vi "Read Config.vi"(6 "wait for reply (T)":bool=TRUE, 8 "error in":errorcluster) -> (0 "error out":errorcluster, 1 "timed out?":bool, 2 "Señal Digital":T1={"Puertos/Pines"="", "Puerto"="DAQSim1", "Pines"=[], "Tiempo de AQ"=0.0, "Tiempo entre AQ"=0.0}, 3 "Señal Analogica":T2={"Canal/Canales"="", "Canal"="DAQSim1", "Canales"=[], "Frecuencia de muestreo"=1000, "Numero de muestras"=1000, "Tiempo de AQ"=0.0})   [LabVIEW 2020, in "Settings.lvlib"]
doc: "Read Digital and Analog info from Data Base\n_____\nCreated using Delacor QMH Event Scripter 6.0.0.121."
uses:
  Settings.lvlib
  Aqcisition/Analog Signal Config.ctl
  Aqcisition/Digital Signal Config.ctl
  Read Config Argument--cluster.ctl
  Read Config (Reply Payload)--cluster.ctl
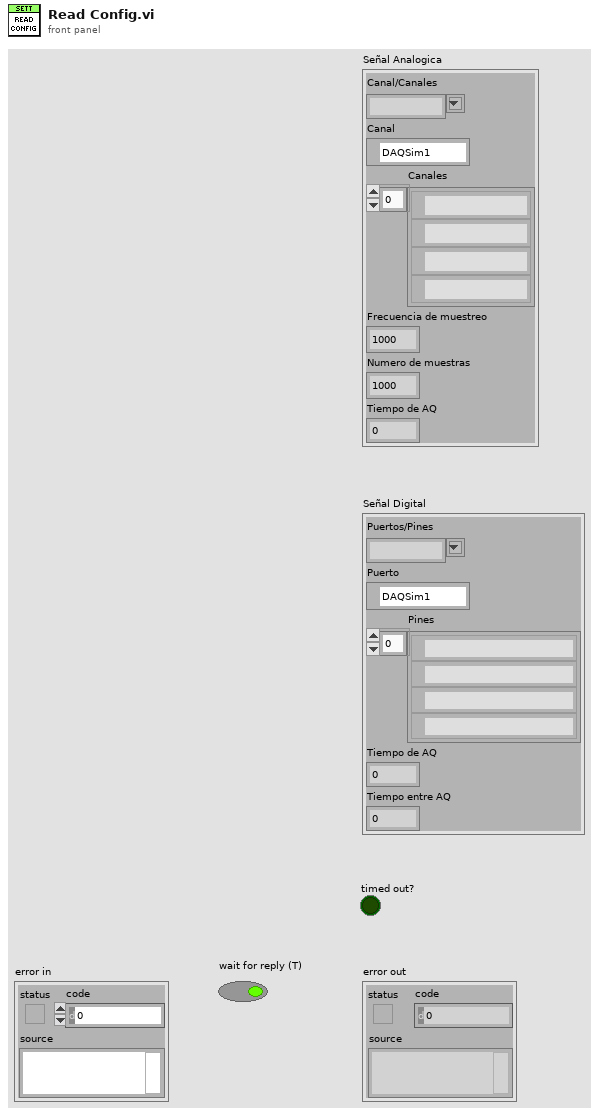
[diagram p1: front panel]
types:
  T1 = typedef "Digital Signal Config.ctl" = cluster{"Puertos/Pines":string, "Puerto":tag, "Pines":tag[], "Tiempo de AQ":dbl, "Tiempo entre AQ":dbl}
  T2 = typedef "Analog Signal Config.ctl" = cluster{"Canal/Canales":string, "Canal":tag, "Canales":tag[], "Frecuencia de muestreo":i32, "Numero de muestras":i32, "Tiempo de AQ":dbl}
  T3 = typedef "Settings.lvlib/Read Config Argument--cluster.ctl" = cluster{"Wait Notifier":refnum<notifier>, "wait for reply":bool}
  T4 = typedef "Settings.lvlib/Request Events--cluster.ctl" = cluster{"Stop Module":refnum<user-event>, "Show Panel":refnum<user-event>, "Hide Panel":refnum<user-event>, "Get Module Execution Status":refnum<user-event>, "Show Diagram":refnum<user-event>, "Save Config":refnum<user-event>, "Read Config":refnum<user-event>, "Save the config":refnum<user-event>, "Cancel config":refnum<user-event>}
  T5 = typedef "Settings.lvlib/Read Config (Reply Payload)--cluster.ctl" = cluster{"Señal Analogica":T2, "Señal Digital":T1, "Read Config_error":errorcluster}
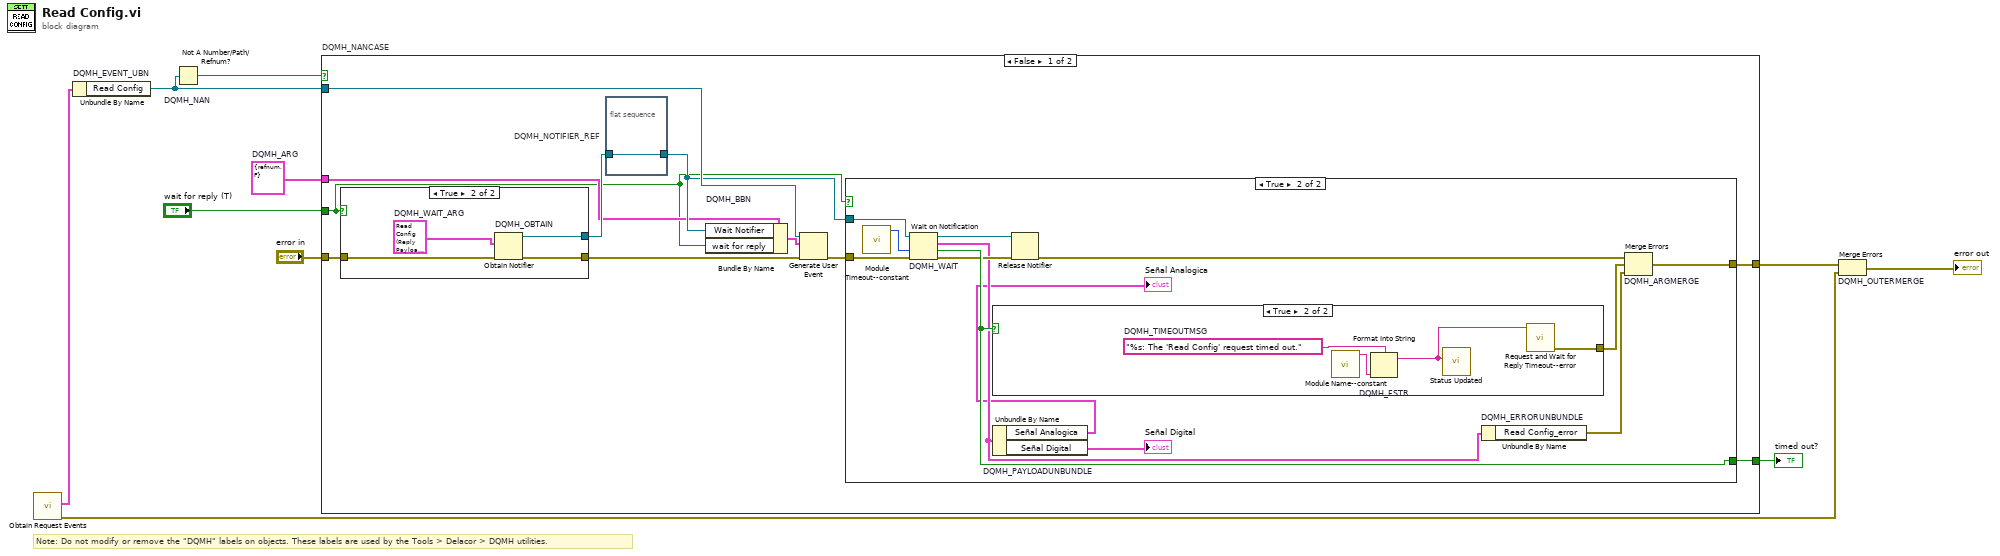
[diagram p0: block diagram]
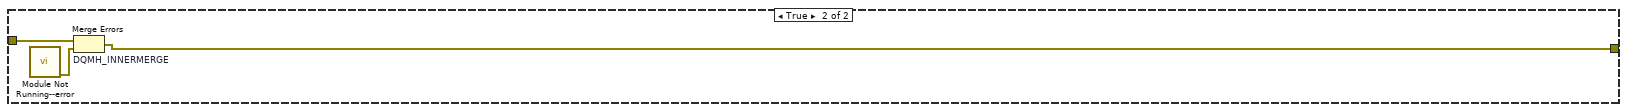
[diagram p5: hidden frame]
diagram:
  w4 = T3 {"Wait Notifier"=refnum, "wait for reply"=FALSE}  # DQMH_ARG
  # "Note: Do not modify or remove the \"DQMH\" labels on objects. These labels are used by the Tools > Delacor > DQMH utilities."
  n1 = call "Obtain Request Events.vi"() -> ("error out"=w2:errorcluster, "Settings Request Events"=w1:T4)  [unwired: 10 in]
  n2 = Unbundle By Name "DQMH_EVENT_UBN"(w1) -> ("Read Config"=w8:refnum<user-event>)
  n3 = Not A Number/Path/Refnum? "DQMH_NAN"(number/path/refnum=w8) -> (NaN/Path/Refnum?=w7:bool)
  n4 = case "DQMH_NANCASE" shown="False" w7 {
    tunnel: "error in" -> [w21 w48]
    tunnel: w8 -> [w19 _]
    tunnel: [w16 w47] -> w5
    tunnel: [w17 _] -> w6
    tunnel: w4 -> [w12 _]
    tunnel: "wait for reply (T)" -> [w11 _]
    frame False {
      n5 = case shown="True" w11 {
        tunnel: w21 -> [w41 w45]
        tunnel: [w41 w44] -> w18
        tunnel: [_ w42] -> w14
        frame False {
        }
        frame True {
          w43 = T5 {"Señal Analogica"={"Canal/Canales"="", "Canal"="DAQSim1", "Canales"=[], "Frecuencia de muestreo"=1000, "Numero de muestras"=1000, "Tiempo de AQ"=0.0}, "Señal Digital"={"Puertos/Pines"="", "Puerto"="DAQSim1", "Pines"=[], "Tiempo de AQ"=0.0, "Tiempo entre AQ"=0.0}, "Read Config_error"={"status"=FALSE, "code"=0, "source"=""}}  # DQMH_WAIT_ARG
          n6 = Obtain Notifier "DQMH_OBTAIN"(notification data type=w43, error in (no error)=w45) -> (notifier out=w42:refnum<notifier>, error out=w44:errorcluster)  [unwired: 2 in, 1 out]
        }
      }
      n7 = flat-sequence "DQMH_NOTIFIER_REF" {
        tunnel: w14 -> [w22]
        tunnel: [w22] -> w13
        frame #0 {
        }
      }
      n8 = Bundle By Name "DQMH_BBN"(cluster=w12, "Wait Notifier"=w13, "wait for reply"=w11) -> (w15:T3)
      n9 = Generate User Event(user event=w19, event data cluster=w15, error in=w18) -> (error out=w20:errorcluster)  [unwired: 1 in, 1 out]
      n10 = case shown="True" w11 {
        tunnel: w20 -> [w23 w36]
        tunnel: w13 -> [_ w35]
        tunnel: [_ w33] -> w17
        tunnel: [w23 w32] -> w16
        frame False {
        }
        frame True {
          n11 = call "Module Timeout--constant.vi"() -> ("Module Timeout"=w26:i32)  [unwired: 11 in]
          n12 = Wait on Notification "DQMH_WAIT"(notifier=w35, timeout in ms (-1)=w26, error in (no error)=w36) -> (notifier out=w34:refnum<notifier>, notification=w27:T5, timed out?=w33:bool, error out=w31:errorcluster)  [unwired: 1 in]
          n13 = case shown="True" w33 {
            tunnel: [_ w38] -> w28
            frame False {
            }
            frame True {
              w40 = "%s: The 'Read Config' request timed out."  # DQMH_TIMEOUTMSG
              n14 = call "Module Name--constant.vi"() -> ("Module Name"=w37:string)  [unwired: 11 in]
              n15 = Format Into String "DQMH_FSTR"(format string=w40, w37) -> (resulting string=w39:string)  [unwired: 2 in, 1 out]
              n16 = call "Status Updated.vi"("Status"=w39) -> ()  [unwired: 10 in, 1 out]
              n17 = call "Request and Wait for Reply Timeout--error.vi"("Error Message"=w39) -> ("error out"=w38:errorcluster)  [unwired: 10 in]
            }
          }
          n18 = Unbundle By Name "DQMH_PAYLOADUNBUNDLE"(w27) -> ("Señal Analogica"=→"Señal Analogica":T2, "Señal Digital"=→"Señal Digital":T1)
          n19 = Release Notifier(notifier=w34, error in (no error)=w31) -> (error out=w30:errorcluster)  [unwired: 1 in, 2 out]
          n20 = Unbundle By Name "DQMH_ERRORUNBUNDLE"(w27) -> ("Read Config_error"=w29:errorcluster)
          n21 = Merge Errors "DQMH_ARGMERGE"(w30, w28, w29) -> (w32:errorcluster)
        }
      }
    }
    frame True {
      n22 = call "Module Not Running--error.vi"() -> ("error out"=w46:errorcluster)  [unwired: 11 in]
      n23 = Merge Errors "DQMH_INNERMERGE"(w48, w46) -> (w47:errorcluster)
    }
  }
  "timed out?" <- w6
  n24 = Merge Errors "DQMH_OUTERMERGE"(w5, w2) -> (→"error out":errorcluster)
